vi "Finalize To Settings.vi"(8 "error in (no error)":errorcluster, 11 "DSF Buffer Converter Transfer Configuration in":refnum<class "Default Buffer Converter Transfer Configuration.lvclass">) -> (0 "error out":errorcluster, 2 "settings":cluster{"key":string, "value":string}[](array[cluster]), 3 "DSF Buffer Converter Transfer Configuration out":refnum<class "Default Buffer Converter Transfer Configuration.lvclass">)   [LabVIEW 2019, in "DSF Core.lvlib" / "Default Buffer Converter Transfer Configuration.lvclass"]
uses:
  Default Buffer Converter Transfer Configuration.lvclass
  Default Buffer Converter Transfer Configuration.lvclass/Default Buffer Converter Transfer Configuration.ctl
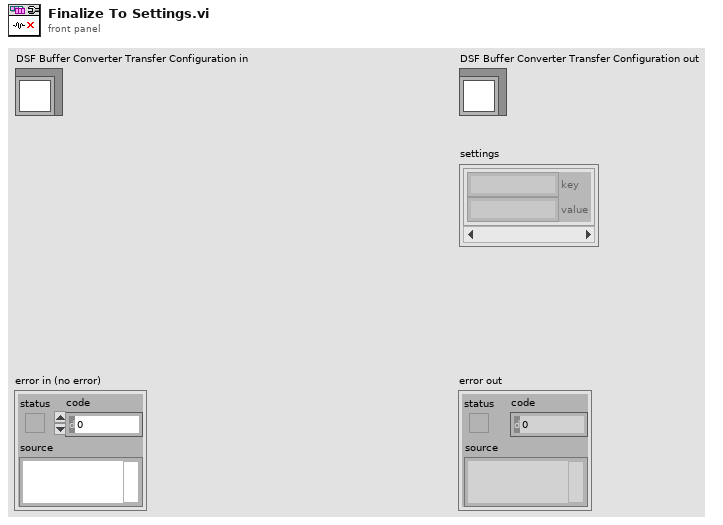
[diagram p1: front panel]
types:
  T1 = typedef "DSF Core.lvlib/DSF Byte Order.ctl" = enum8{"big-endian", "little-endian"}
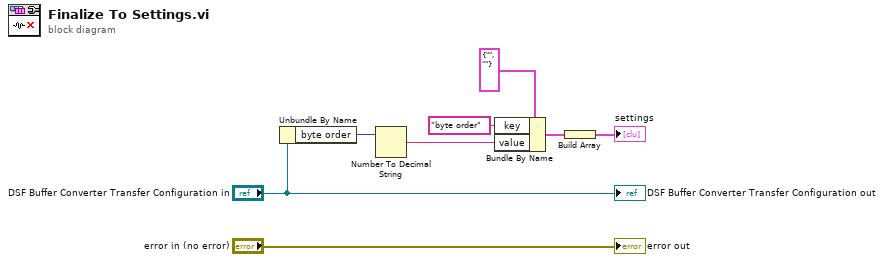
[diagram p0: block diagram]
diagram:
  n1 = Unbundle By Name("DSF Buffer Converter Transfer Configuration in") -> ("byte order"=w4:T1)
  n2 = Number To Decimal String(number=w4) -> (decimal integer string=w3:string)  [unwired: 1 in]
  n3 = Bundle By Name(cluster=cluster{"key":string, "value":string} {"key"="", "value"=""} ("settings"), "key"="byte order", "value"=w3) -> (w2:cluster{"key":string, "value":string})
  n4 = Build Array(w2) -> (→"settings":cluster{"key":string, "value":string}[])
  "error out" <- "error in (no error)"
  "DSF Buffer Converter Transfer Configuration out" <- "DSF Buffer Converter Transfer Configuration in"
